vi "Delete CSM-VI.vi"(6 "Config Path":path, 8 "error in (no error)":errorcluster, 11 "CSM Name":string) -> (0 "error out":errorcluster)   [LabVIEW 2017, in "CSM-Helper API with lvcsm Support.lvlib"]
uses:
  CSM-Helper API with lvcsm Support.lvlib
  <vilib>/Utility/config.llb/Read Key (String).vi
  <vilib>/Utility/config.llb/NI_LVConfig.lvlib
  lvcsmFile/lvcsm File Support.lvlib
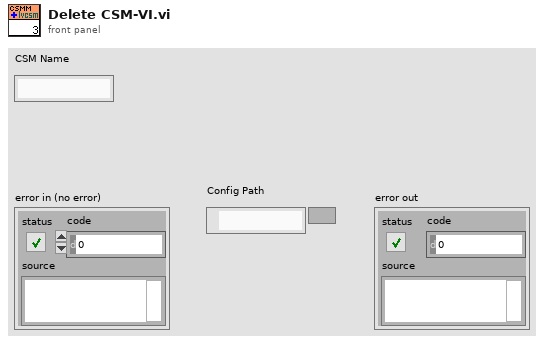
[diagram p1: front panel]
types:
  T1 = typedef "NI_LVConfig.lvlib/Config Data RefNum.ctl" = refnum<k1>
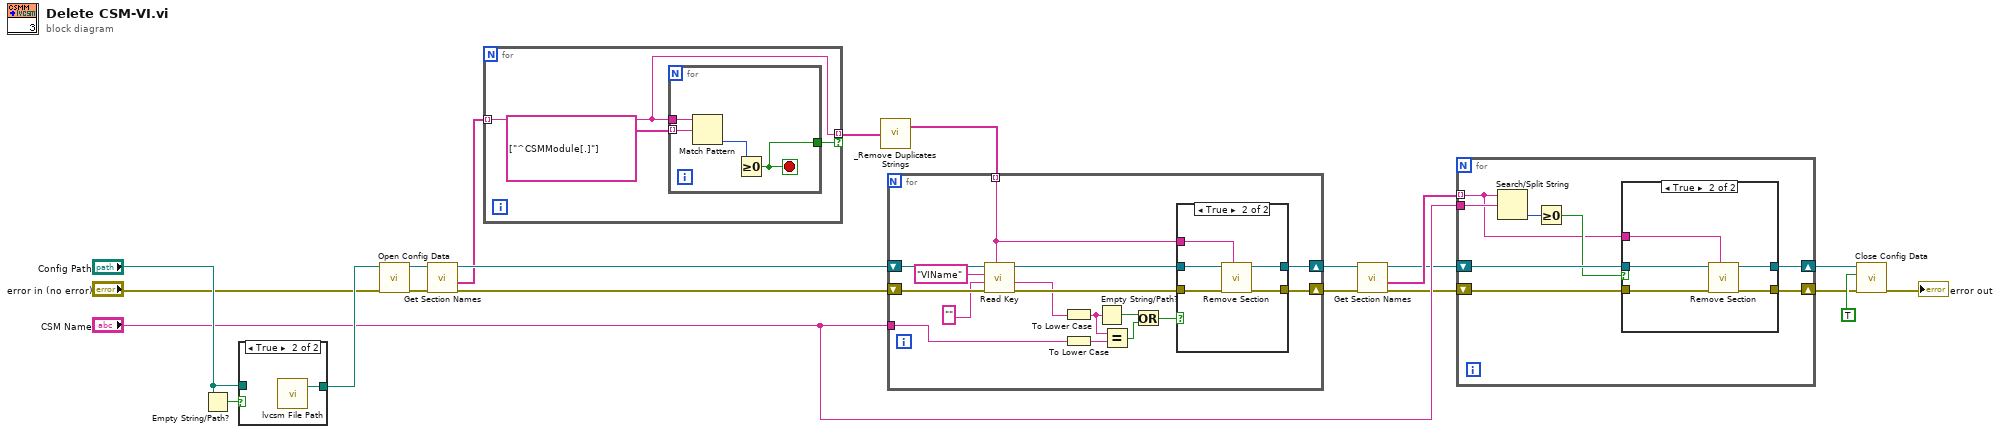
[diagram p0: block diagram]
diagram:
  n1 = Empty String/Path?(string/path="Config Path") -> (empty?=w19:bool)
  n2 = case shown="True" w19 {
    tunnel: [w22 w23] -> w21
    tunnel: "Config Path" -> [w22 _]
    frame False {
    }
    frame True {
      n3 = call "lvcsm File Path.vi"() -> ("Appended Path"=w23:path)  [unwired: 3 in]
    }
  }
  n4 = call <vilib>:"Open Config Data.vi"("error in (no error)"="error in (no error)", "configuration file path"=w21) -> ("error out"=w15:errorcluster, "refnum"=w14:T1)  [unwired: 7 in, 1 out]
  n5 = call <vilib>:"Get Section Names.vi"("error in (no error)"=w15, "refnum"=w14) -> ("error out"=w13:errorcluster, "section names"=w10:string[], "refnum out"=w12:T1)  [unwired: 7 in]
  n6 = for {
    tunnel: w10 -> [w24] mode=indexing
    tunnel: [w24] -> w11 mode=indexing if=w25
    n7 = for {
      tunnel: w24 -> [w30]
      tunnel: string[] ["^CSMModule[.]"] ("regular expression") -> [w29] mode=indexing
      tunnel: [w27] -> w25
      stop <- w27 stop-if-true
      n8 = Match Pattern(string=w30, regular expression=w29) -> (offset past match=w28:i32)  [unwired: 1 in, 3 out]
      n9 = Greater Or Equal To 0?(x=w28) -> (x >= 0?=w27:bool)
    }
  }
  n10 = call "_Remove Duplicates Strings.vi"("Input Array"=w11) -> ("Output Array"=w9:string[])  [unwired: 1 out]
  n11 = for {
    tunnel: w9 -> [w38] mode=indexing
    shift-right: [w40] -> w8
    shift-left: w13 -> [w46]
    shift-right: [w39] -> w7
    shift-left: w12 -> [w45]
    tunnel: "CSM Name" -> [w31]
    n12 = call-poly <vilib>:"Read Key.vi"("section"=w38, "error in (no error)"=w46, "default value"="" ("key"), "key"="VIName", "refnum"=w45) -> ("error out"=w41:errorcluster, "value"=w37:string, "refnum out"=w42:T1)  [unwired: 3 in, 1 out]
    n13 = To Lower Case(string=w37) -> (all lower case string=w32:string)
    n14 = To Lower Case(string=w31) -> (all lower case string=w33:string)
    n15 = Empty String/Path?(string/path=w32) -> (empty?=w36:bool)
    n16 = Equal?(x=w32, y=w33) -> (x = y?=w34:bool)
    n17 = Or(x=w36, y=w34) -> (x .or. y?=w35:bool)
    n18 = case shown="True" w35 {
      tunnel: w42 -> [w48 w53]
      tunnel: w41 -> [w47 w52]
      tunnel: [w47 w51] -> w40
      tunnel: [w48 w50] -> w39
      tunnel: w38 -> [_ w49]
      frame False {
      }
      frame True {
        n19 = call <vilib>:"Remove Section.vi"("section"=w49, "error in (no error)"=w52, "refnum"=w53) -> ("error out"=w51:errorcluster, "refnum out"=w50:T1)  [unwired: 6 in, 1 out]
      }
    }
  }
  n20 = call <vilib>:"Get Section Names.vi"("error in (no error)"=w8, "refnum"=w7) -> ("error out"=w4:errorcluster, "section names"=w6:string[], "refnum out"=w3:T1)  [unwired: 7 in]
  n21 = for {
    tunnel: w6 -> [w54] mode=indexing
    tunnel: "CSM Name" -> [w61]
    shift-right: [w57] -> w2
    shift-left: w4 -> [w60]
    shift-right: [w58] -> w1
    shift-left: w3 -> [w59]
    n22 = Search/Split String(string=w54, search string/char (-)=w61) -> (offset of match=w56:i32)  [unwired: 1 in, 2 out]
    n23 = Greater Or Equal To 0?(x=w56) -> (x >= 0?=w55:bool)
    n24 = case shown="True" w55 {
      tunnel: w60 -> [w62 w68]
      tunnel: w59 -> [w63 w67]
      tunnel: [w63 w66] -> w58
      tunnel: [w62 w65] -> w57
      tunnel: w54 -> [_ w64]
      frame False {
      }
      frame True {
        n25 = call <vilib>:"Remove Section.vi"("section"=w64, "error in (no error)"=w68, "refnum"=w67) -> ("error out"=w65:errorcluster, "refnum out"=w66:T1)  [unwired: 6 in, 1 out]
      }
    }
  }
  n26 = call <vilib>:"Close Config Data.vi"("error in (no error)"=w2, "write file if changed (T)"=TRUE, "refnum"=w1) -> ("error out"=→"error out":errorcluster)  [unwired: 7 in, 1 out]
